vi "数据缓冲.vi"(8 "读取":bool, 9 "Y轴距离":dbl, 10 "X轴距离":dbl, 11 "清零":bool) -> (2 "Y轴":dbl[](array[numeric]), 3 "X轴":dbl[](array[numeric]))   [LabVIEW 2011]
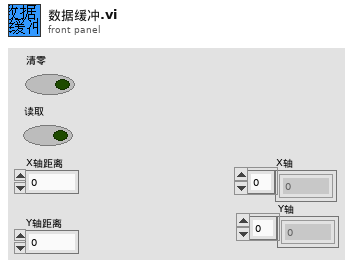
[diagram p1: front panel]
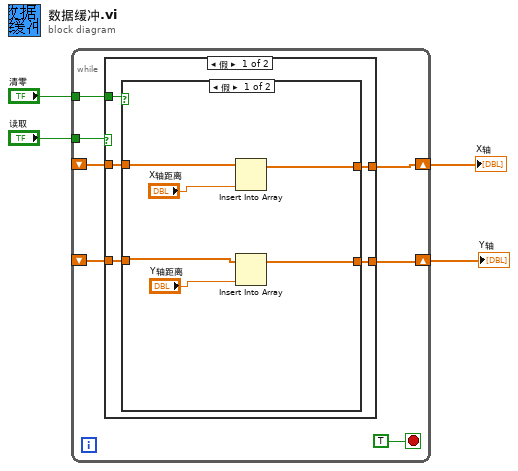
[diagram p0: block diagram]
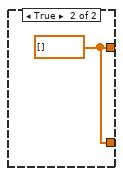
[diagram p2: hidden frame]
diagram:
  n1 = while {
    tunnel: "清零" -> [w10]
    shift-right: [w8] -> w3
    shift-left: _ -> [w9]
    shift-right: [w6] -> w2
    shift-left: _ -> [w7]
    tunnel: "读取" -> [w5]
    stop <- TRUE stop-if-true
    n2 = case shown="假" w5 {
      tunnel: w10 -> [w16 _]
      tunnel: w9 -> [w15 w25]
      tunnel: [w14 w25] -> w8
      tunnel: w7 -> [w13 w24]
      tunnel: [w12 w24] -> w6
      frame False {
        n3 = case shown="假" w16 {
          tunnel: w15 -> [w22 _]
          tunnel: [w21 w23] -> w14
          tunnel: w13 -> [w19 _]
          tunnel: [w18 w23] -> w12
          frame False {
            n4 = Insert Into Array(array=w22, new element="X轴距离") -> (w21:dbl[])  [unwired: 1 in]
            n5 = Insert Into Array(array=w19, new element="Y轴距离") -> (w18:dbl[])  [unwired: 1 in]
          }
          frame True {
            w23 = dbl[] []
          }
        }
      }
      frame True {
      }
    }
  }
  "X轴" <- w3
  "Y轴" <- w2
